vi "Tree Parameters.vi"() -> (2 "Font Size":i32, 3 "Row Height":i32)   [LabVIEW 2023]
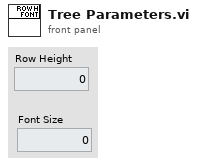
[diagram p1: front panel]
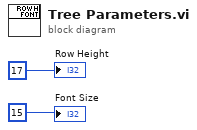
[diagram p0: block diagram]
diagram:
  "Row Height" <- 17
  "Font Size" <- 15
